vi "Pracownia4v2niecała.vi"() -> ()   [LabVIEW 2023]
uses:
  eb685d7e-d23d-492b-ba15-63d608dacec0.vi
  <vilib>/Array/Sort 2D Array - Pop Stack.vi
  <vilib>/Array/Sort 2D Array - Push Stack.vi
  eb685d7e-d23d-492b-ba15-63d608dacec0.vi/269d4b3b-47f5-49e3-8884-44851e4dd9d5.vi
  eb685d7e-d23d-492b-ba15-63d608dacec0.vi/6d99389c-673d-4efb-bf33-19b32bcf4cf8.vi
panel:
  out "nr iteracji":i32
  in  "stop":bool
  out "sorted 2D array":dbl[][](array[numeric])
  out "Array with sorted rows":dbl[][](array[numeric])
  out "element (9,9)":dbl
  out "last generated value":dbl
  out "Array":dbl[][](array[numeric])
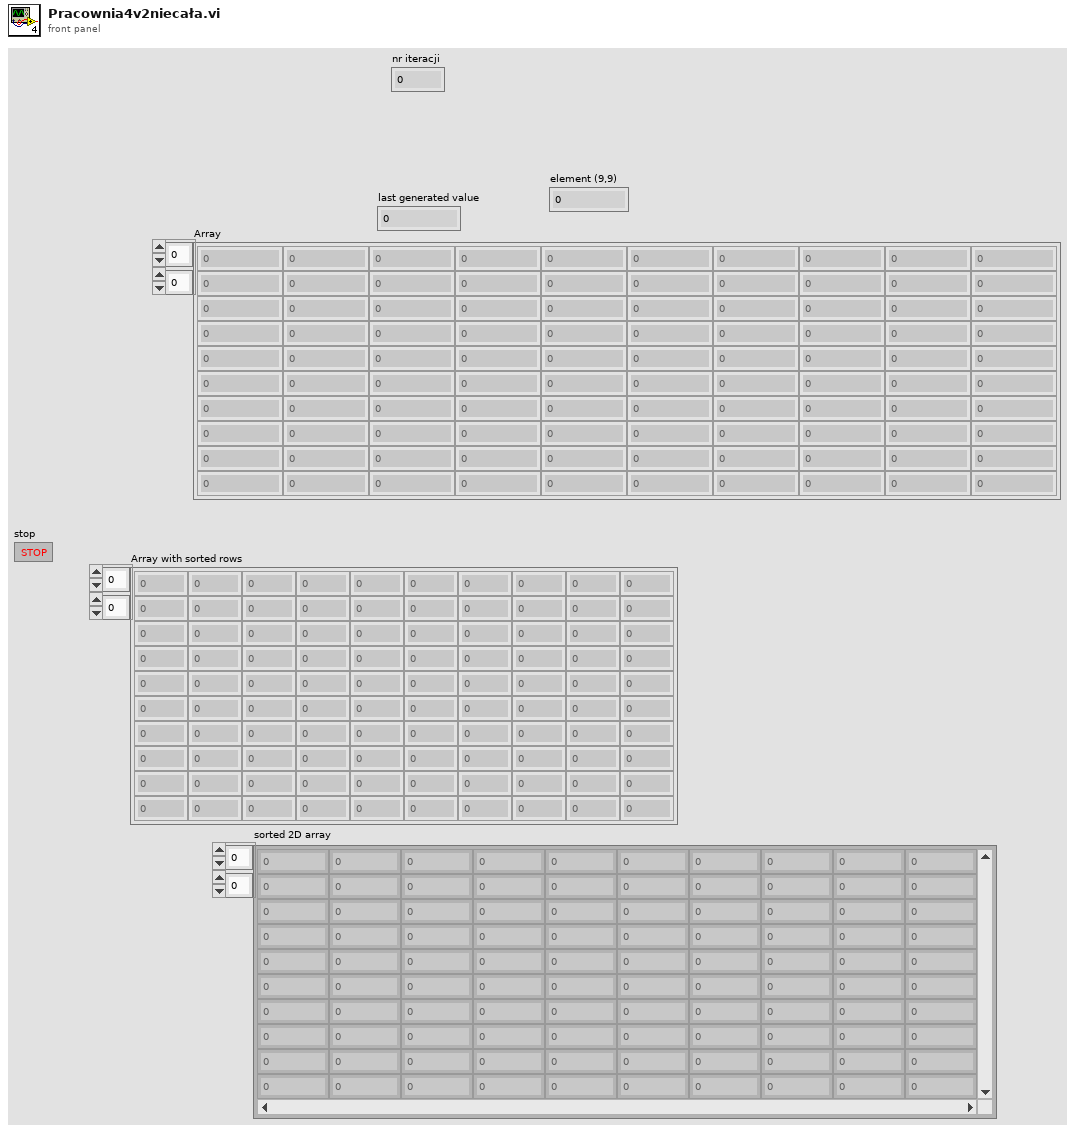
[diagram p1: front panel]
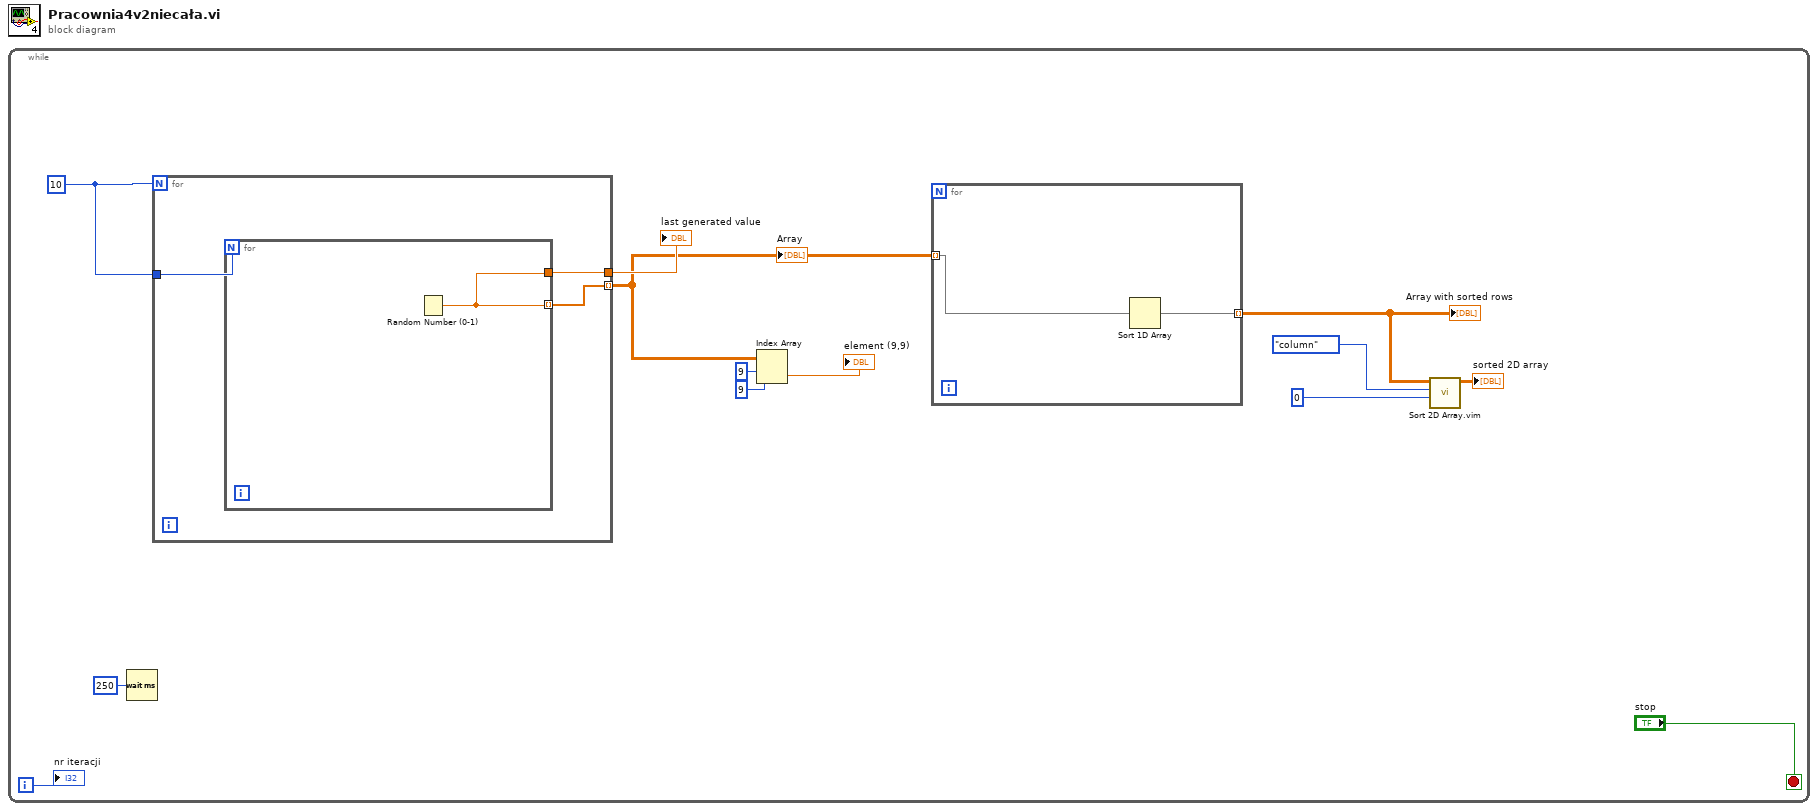
[diagram p0: block diagram]
diagram:
  n1 = while {
    i -> [w2]
    stop <- "stop" stop-if-true
    w13 = 10
    n2 = Wait (ms)(milliseconds to wait=u32 250) -> ()  [unwired: 1 out]
    n3 = for {
      N: w13 -> [_]
      tunnel: [w18] -> w8 mode=indexing
      tunnel: w13 -> [w17]
      tunnel: [w16] -> w12
      n4 = for {
        N: w17 -> [_]
        tunnel: [w19] -> w18 mode=indexing
        tunnel: [w19] -> w16
        n5 = Random Number (0-1)() -> (number: 0 to 1=w19:dbl)
      }
    }
    "Array" <- w8
    "last generated value" <- w12
    n6 = Index Array(array=w8, index (row)=9, index (col)=9 ("disabled index (col)")) -> (element=→"element (9,9)":dbl)
    n7 = for {
      tunnel: w8 -> [w15] mode=indexing
      tunnel: [w14] -> w5 mode=indexing
      n8 = Sort 1D Array(array=w15) -> (sorted array=w14:dbl[])
    }
    "Array with sorted rows" <- w5
    n9 = call "Sort 2D Array.vim"("index"=0, "dimension to index (column)"=enum16{"column", "row"}."column", "2D array"=w5) -> ("sorted 2D array"=→"sorted 2D array":dbl[][])  [unwired: 7 in, 1 out]
    "nr iteracji" <- w2
  }
